vi "Window Comparison.vi"() -> ()   [LabVIEW 2020]
doc: "This example demonstrates the importance of using windows when performing spectral analysis on signals which contain multiple frequencies.\n\nThe effect of different types of window functions is shown in the frequency domain. With no window function used, Sine Wave 2 buries the low amplitude Sine Wave 1. Using the Hanning Window (Window 2), the smaller signal can be detected."
uses:
  <vilib>/Analysis/0measdsp.llb/Scaled Time Domain Window (DBL).vi
  <vilib>/Analysis/NI_AALBase.lvlib
  <vilib>/Analysis/NI_AALPro.lvlib
panel:
  in  "window 1":u32(ring) items=["Rectangle"=0, "Hanning"=1, "Hamming"=2, "Blackman-Harris"=3, "Exact Blackman"=4, "Blackman"=5, "Flat Top"=6, "4 Term B-Harris "=7, "7 Term B-Harris"=8, "Low Sidelobe"=9, "Blackman Nuttall"=11, "Triangle"=30, "Bartlett-Hanning"=31, "Bohman"=32, "Parzen"=33, "Welch"=34, "Kaiser"=60, "Dolph-Chebyshev"=61, "Gaussian"=62]
  in  "window 2":u32(ring)=1 items=["Rectangle"=0, "Hanning"=1, "Hamming"=2, "Blackman-Harris"=3, "Exact Blackman"=4, "Blackman"=5, "Flat Top"=6, "4 Term B-Harris "=7, "7 Term B-Harris"=8, "Low Sidelobe"=9, "Blackman Nuttall"=11, "Triangle"=30, "Bartlett-Hanning"=31, "Bohman"=32, "Parzen"=33, "Welch"=34, "Kaiser"=60, "Dolph-Chebyshev"=61, "Gaussian"=62]
  in  "frequency 2":dbl(slide)=81.82 scale=0.0..100.0
  in  "amplitude 2":dbl=0.001 format="%#.6g"
  in  "amplitude 1":dbl=1.0 format="%#.6g"
  in  "frequency 1":dbl(slide)=60.5 scale=0.0..100.0
  in  "Stop":bool
  out "Frequency Domain":dbl[][](graph)
  out "Time Domain":dbl[](graph)
  # "Overview: Explore the effects of different types of window functions in the frequency domain. \nRequirements: LabVIEW Full Development System\nInstructions: \n1. Run the VI. Notice that with window 1 set to \"Rectangle\", tone 1 buries the lower-amplitude tone 2.  \n2. Change window 1 and/or window 2 to compare different window shapes.\n3. Change the amplitude and frequency values to see how different signals are affected by windowing.\n4. Click Stop to stop the VI."
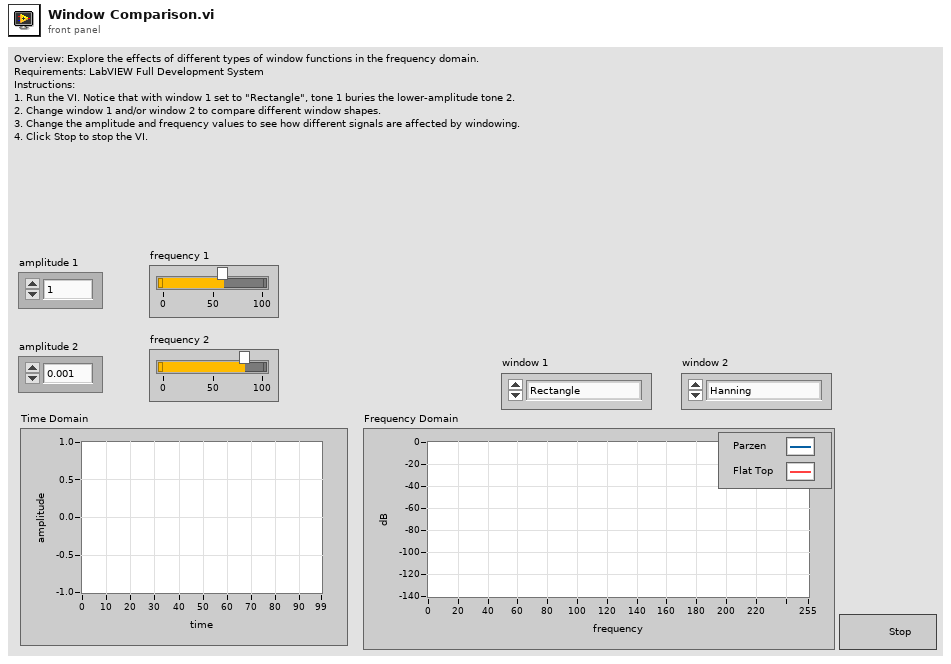
[diagram p1: front panel]
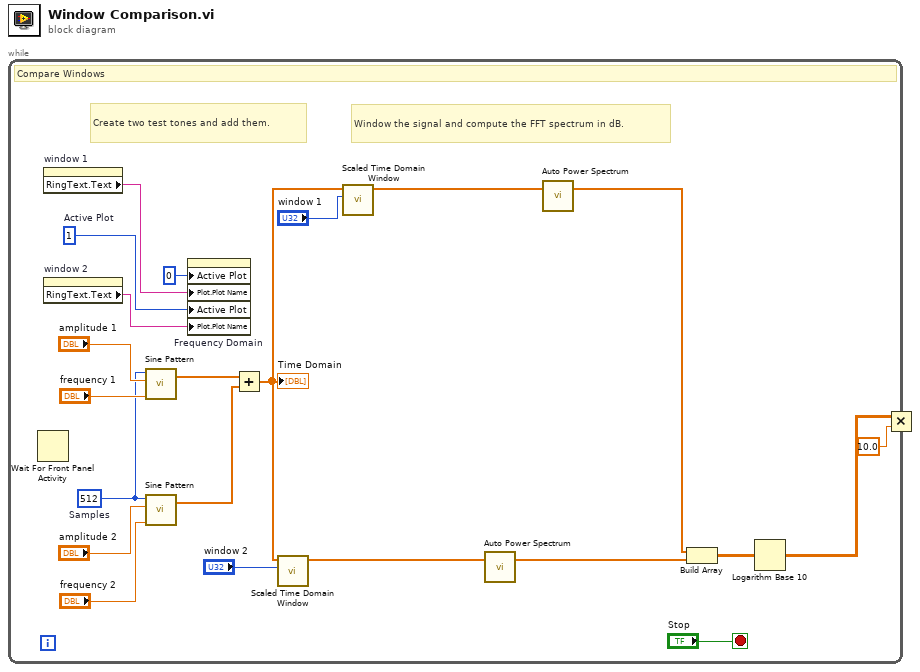
[diagram p0: block diagram]
diagram:
  n1 = while {
    stop <- "Stop" stop-if-true
    w2 = 512  # Samples
    w8 = u32 1  # Active Plot
    # "Window the signal and compute the FFT spectrum in dB."
    # "Create two test tones and add them."
    # "Compare Windows"
    n2 = Wait For Front Panel Activity() -> ()  [unwired: 3 in, 1 out]
    n3 = property on="window 1" class="Ring (strict)"() -> ("RingText.Text"=w6:string)  [unwired: 2 in, 2 out]
    n4 = property on="window 2" class="Ring (strict)"() -> ("RingText.Text"=w5:string)  [unwired: 2 in, 2 out]
    n5 = call <vilib>:"Sine Pattern.vi"("cycles"="frequency 1", "amplitude"="amplitude 1", "samples"=w2) -> ("Sinusoidal Pattern"=w22:dbl[])  [unwired: 1 in, 1 out]
    n6 = call <vilib>:"Sine Pattern.vi"("cycles"="frequency 2", "amplitude"="amplitude 2", "samples"=w2) -> ("Sinusoidal Pattern"=w21:dbl[])  [unwired: 1 in, 1 out]
    n7 = property on="Frequency Domain" class="WFGraph (strict)"("Active Plot"=u32 0, "Plot.Plot Name"=w6, "Active Plot"=w8, "Plot.Plot Name"=w5) -> ()  [unwired: 2 in, 2 out]
    n8 = Add(x=w22, y=w21) -> (x+y=w10:dbl[])
    "Time Domain" <- w10
    n9 = call-poly <vilib>:"Scaled Time Domain Window.vi"("window"="window 2", "X"=w10) -> ("Windowed X"=w11:dbl[])  [unwired: 7 in, 2 out]
    n10 = call-poly <vilib>:"Scaled Time Domain Window.vi"("window"="window 1", "X"=w10) -> ("Windowed X"=w12:dbl[])  [unwired: 7 in, 2 out]
    n11 = call <vilib>:"Auto Power Spectrum.vi"("Signal (V)"=w11) -> ("Power Spectrum (V^2 rms)"=w13:dbl[])  [unwired: 1 in, 1 out]
    n12 = call <vilib>:"Auto Power Spectrum.vi"("Signal (V)"=w12) -> ("Power Spectrum (V^2 rms)"=w14:dbl[])  [unwired: 1 in, 1 out]
    n13 = Build Array "Build Array"(w14, w13) -> (w19:dbl[][])
    n14 = Logarithm Base 10(1:w19) -> (0:w20:dbl[][])
    n15 = Multiply(x=w20, y=10.0) -> (x*y=→"Frequency Domain":dbl[][])
  }
